vi "python.vi"() -> ()   [LabVIEW 2018]
panel:
  in  "정지":bool
  out "반환값":string
  out "에러 출력":errorcluster caption="에러 1"
  in  "function_1":string
  in  "1st module":path
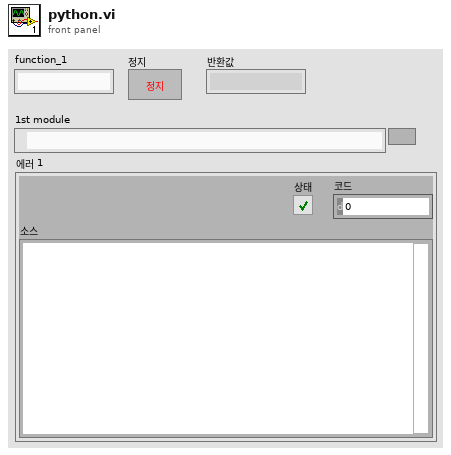
[diagram p1: front panel]
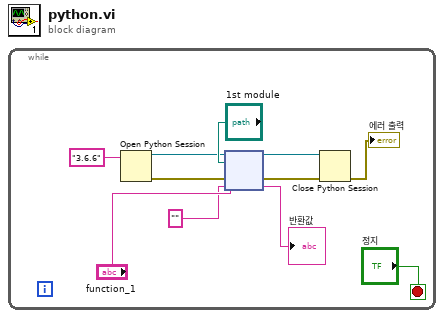
[diagram p0: block diagram]
diagram:
  n1 = while {
    stop <- "정지" stop-if-true
    n2 = Open Python Session(python version="3.6.6" ("Python 버전")) -> (session out=w7:refnum<k35>, error out=w5:errorcluster)  [unwired: 2 in]
    n3 = node(w7, "1st module", "function_1", w5, "") -> (w10:refnum<k35>, w6:errorcluster, →"반환값":string)  [unwired: 2 out]
    n4 = Close Python Session(session in=w10, error in=w6) -> (11:→"에러 출력":errorcluster)
  }
